vi "Compile with Context.vi"(6 "Loader":refnum<class "Loader.lvclass">, 7 "Data":refnum<class "Datum.lvclass">=refnum, 8 "Error In":errorcluster, 10 "Context In":refnum<class "Context.lvclass">, 11 "Input":string) -> (0 "Error Out":errorcluster, 3 "Output":string)   [LabVIEW 2018, in "Toolkit.lvlib"]
doc: "Compiles a Mustache template using the supplied data and their types to control the rendering process. The type fo data for each tag and key determines the rendering behavior of the node in the syntax tree, so LabVIEW classes are provided to convert LabVIEW values and represent the different data types.\n\n<b>Input</b> - A logic-free Mustache template as a string that will be compiled, or rendered, to the output based on the data provided.\n\n<B>Data</B> - Mustache data represented either as an array of key-value pairs, an array of key-value string clusters, or a generic Datum object. The rendering of a Mustache template is dependent on the existence and type of data provided at compilation.\n\n<B>Loader</B> - Responsible for importing, or including, other Mustache templates within the root template.\n\n<B>Output</B> - A string representing the completely lexed, parsed, and rendered Mustache template based on the supplied data's types and values."
uses:
  Toolkit.lvlib
  Data/Datum/Datum.lvclass
  Data/Map/Map.lvclass
  Low-Level/Loaders/Loader/Loader.lvclass
  Low-Level/Context/Context.lvclass
  Low-Level/Support/Lex String.vi
  Low-Level/Support/Render to String.vi
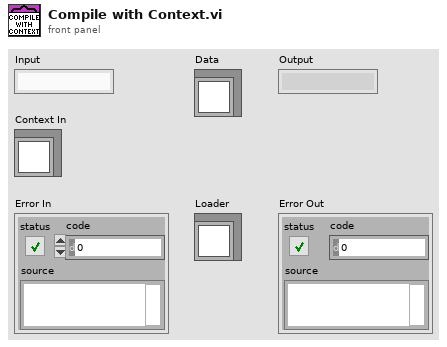
[diagram p1: front panel]
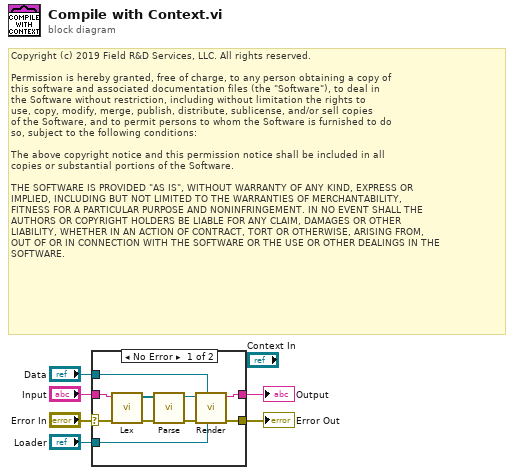
[diagram p0: block diagram]
diagram:
  # "Copyright (c) 2019 Field R&D Services, LLC. All rights reserved.\n\nPermission is hereby granted, free of charge, to any person obtaining a copy of\nthis software and associated documentation files (the \"Software\"), to deal in\nthe Software without restriction, including without limitation the rights to\nuse, copy, modify, merge, publish, distribute, sublicense, and/or sell copies\nof the Software, and to permit persons to whom the Software is furnished to do\nso, subject to the following conditions:\n\nThe above copyright notice and this permission notice shall be included in all\ncopies or substantial portions of the Software.\n\nTHE SOFTWARE IS PROVIDED \"AS IS\", WITHOUT WARRANTY OF ANY KIND, EXPRESS OR\nIMPLIED, INCLUDING BUT NOT LIMITED TO THE WARRANTIES OF MERCHANTABILITY,\nFITNESS FOR A PARTICULAR PURPOSE AND NONINFRINGEMENT. IN NO EVENT SHALL THE\nAUTHORS OR COPYRIGHT HOLDERS BE LIABLE FOR ANY CLAIM, DAMAGES OR OTHER\nLIABILITY, WHETHER IN AN ACTION OF CONTRACT, TORT OR OTHERWISE, ARISING FROM,\nOUT OF OR IN CONNECTION WITH THE SOFTWARE OR THE USE OR OTHER DEALINGS IN THE\nSOFTWARE."
  n1 = case shown="No Error" "Error In" {
    selector: "Error In" -> [w10 w17]
    tunnel: [w13 w17] -> w6
    tunnel: "Input" -> [w9 w18]
    tunnel: [w12 w18] -> w4
    tunnel: "Data" -> [w11 _]
    tunnel: "Loader" -> [w7 _]
    frame No Error {
      n2 = call-poly "Lex.vi"("Error In"=w10, "Input"=w9) -> ("Error Out"=w8:errorcluster, "Tokens"=w16:refnum<class "Token.lvclass">[])  [unwired: 8 in]
      n3 = call "Parse.vi"("Error In"=w8, "Tokens"=w16) -> ("Error Out"=w14:errorcluster, "Abstract Syntax Tree"=w15:refnum<class "Root.lvclass">)  [unwired: 8 in]
      n4 = call-poly "Render.vi"("Loader"=w7, "Data"=w11, "Error In"=w14, "Abstract Syntax Tree"=w15) -> ("Error Out"=w13:errorcluster, "Output"=w12:string)  [unwired: 6 in]
    }
    frame Error {
    }
  }
  "Error Out" <- w6
  "Output" <- w4
